vi "Write Analogue.vi"(8 "error in (no error)":errorcluster, 9 "output":bool, 10 "Channel index":i32, 11 "Abstract Fgen":refnum<class "Fgen Instrument.lvclass">) -> (0 "error out":errorcluster, 2 "Success?":bool=TRUE, 3 "Abstract Fgen out":refnum<class "Fgen Instrument.lvclass">)   [LabVIEW 2025, in "Fgen.lvlib" / "Fgen Instrument.lvclass"]
uses:
  Fgen Instrument.lvclass
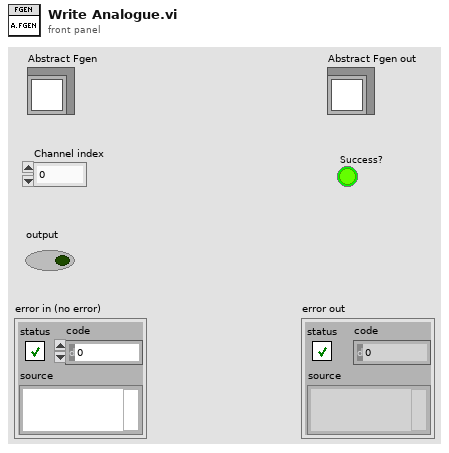
[diagram p1: front panel]
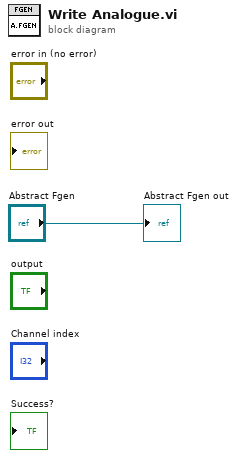
[diagram p0: block diagram]
diagram:
  "Abstract Fgen out" <- "Abstract Fgen"
